vi "ImageBlock_64to32__ (子VI).vi"(1 "8-bit pixmap":u8[][](array[numeric])) -> (0 "数组":u8[][][](array[numeric]))   [LabVIEW 2018]
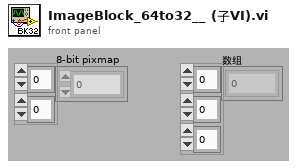
[diagram p1: front panel]
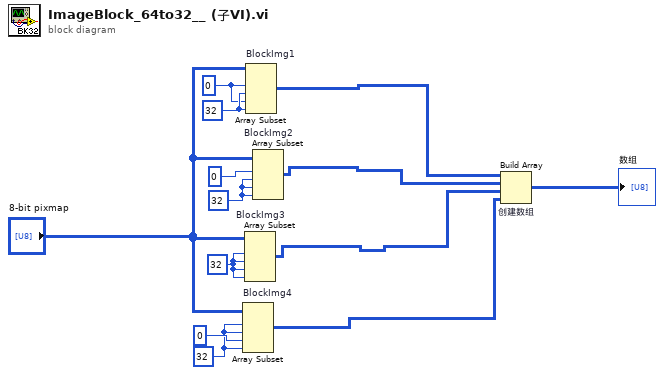
[diagram p0: block diagram]
diagram:
  w6 = 32
  w8 = 32
  w10 = 32
  w12 = 32
  w11 = 0
  n1 = Array Subset "BlockImg4"(array="8-bit pixmap", index (row)=w6, length (row)=w6, index (col)=0, length (col)=w6) -> (w4:u8[][])
  n2 = Array Subset "BlockImg3"(array="8-bit pixmap", index (row)=w8, length (row)=w8, index (col)=w8, length (col)=w8) -> (w3:u8[][])
  n3 = Array Subset "BlockImg1"(array="8-bit pixmap", index (row)=w11, length (row)=w12, index (col)=w11, length (col)=w12) -> (w1:u8[][])
  n4 = Array Subset "BlockImg2"(array="8-bit pixmap", index (row)=0, length (row)=w10, index (col)=w10, length (col)=w10) -> (w2:u8[][])
  n5 = Build Array "创建数组"(w1, w2, w3, w4) -> (→"数组":u8[][][])
